vi "CODMn测量数据储存.vi"   [LabVIEW 2016, in "斯坦道CODMn新电路板.lvlib"]
types:
  T1 = enum16{"空闲", "水样测试", "标样核查", "零点核查", "跨度核查", "空白测试", "平行样测试", "加标回收", "空白校准", "标样校准"}
  T2 = enum16{"水样测试", "标样核查", "跨度核查", "零点核查", "空白测试", "平行样测试", "加标回收", "空白校准", "标样校准"}
  T3 = cluster{"时间标识":timestamp, "监测值":sgl, "单位":u16, "数据标识":string, "因子编码":u32, "标样参考值":sgl, "A":sgl, "B":sgl, "K":sgl, "终点滴定数":sgl, "环境温度":sgl, "环境湿度":sgl, "量程":sgl, "加热实时温度":sgl, "X0":sgl, "X^2":sgl, "X":sgl, "B 2":sgl, "跨度值":sgl}
  T4 = enum16{"维护数据", "水样测试", "标样核查", "零点核查", "跨度核查", "空白测试", "平行样测试", "加标回收", "空白校准", "标样校准", "初始化（清洗）"}
  T5 = cluster{"运行模式":enum16{"维护模式", "常规模式", "应急模式", "质控模式"}, "质控频次":enum16{"关闭", "每天", "星期一", "星期二", "星期三", "星期四", "星期五", "星期六", "星期日"}, "空白核查时间":u16, "跨度核查时间":u16, "测量间隔":u16}
  T6 = cluster{"系统时间":timestamp, "工作状态":u16, "测量模式":enum16{"待机", "连续模式", "周期模式", "定点模式", "受控模式", "手动模式"}, "告警代码":u16, "故障代码":u16, "日志代码":u16, "软件版本":u16, "A":sgl, "B":sgl, "K":sgl, "当前滴定数":sgl, "T":sgl, "H":sgl, "id":u16, "flowid":u16, "量程":u16, "加热实时温度":sgl, "当前ORP值":sgl, "运行时间":sgl, "当前步骤剩余时间":sgl, "结束滴定数":sgl, "注射泵保温温度":sgl, "匹配滴定数X0":u16, "X^2":sgl, "X":sgl, "B 2":sgl}
  T7 = cluster{"因子编码":u32, "单位":u16, "标样参考值":sgl, "水样数据时间":timestamp, "水样实测值":sgl, "水样数据标识":string, "标样数据时间":timestamp, "标样实测值":sgl, "标样数据标识":string, "空白数据时间":timestamp, "空白实测值":sgl, "空白数据标识":string, "零点核查数据时间":timestamp, "零点核查实测值":sgl, "零点核查数据标识":string, "跨度核查数据时间":timestamp, "跨度核查实测值":sgl, "跨度核查数据标识":string, "加标回收数据时间":timestamp, "加标回收实测值":sgl, "加标回收数据标识":string, "平行样数据时间":timestamp, "平行样实测值":sgl, "平行样数据标识":string, "F0":sgl, "F1":sgl, "F2":sgl, "F3":sgl, "F4":sgl, "F5":sgl, "F6":sgl, "F7":sgl, "温度":sgl, "湿度":sgl, "X值":sgl, "fidrange":u16}
  T8 = cluster{"跨度值":dbl, "零点标准液浓度":dbl, "跨度标准液浓度":dbl, "标准液标准浓度":dbl}
  T9 = cluster{"公式":cluster{"X^2":dbl, "X":dbl, "B":dbl}, "校准":cluster{"校准？":bool, "校准点1-5":u16, "校准浓度":dbl}}
  T10 = cluster{"测量量程":sgl, "测量检出限":sgl, "测量精度":sgl, "测量间隔":sgl, "消解温度":sgl, "消解时长":sgl, "三项式系数":sgl, "二次多项式系数":sgl, "曲线斜率":sgl, "曲线截距":sgl, "线性相关系数":sgl, "空白校准时间":timestamp, "标样校准时间":timestamp, "测量信号值":sgl, "稀释倍数":sgl, "量程系数":sgl}
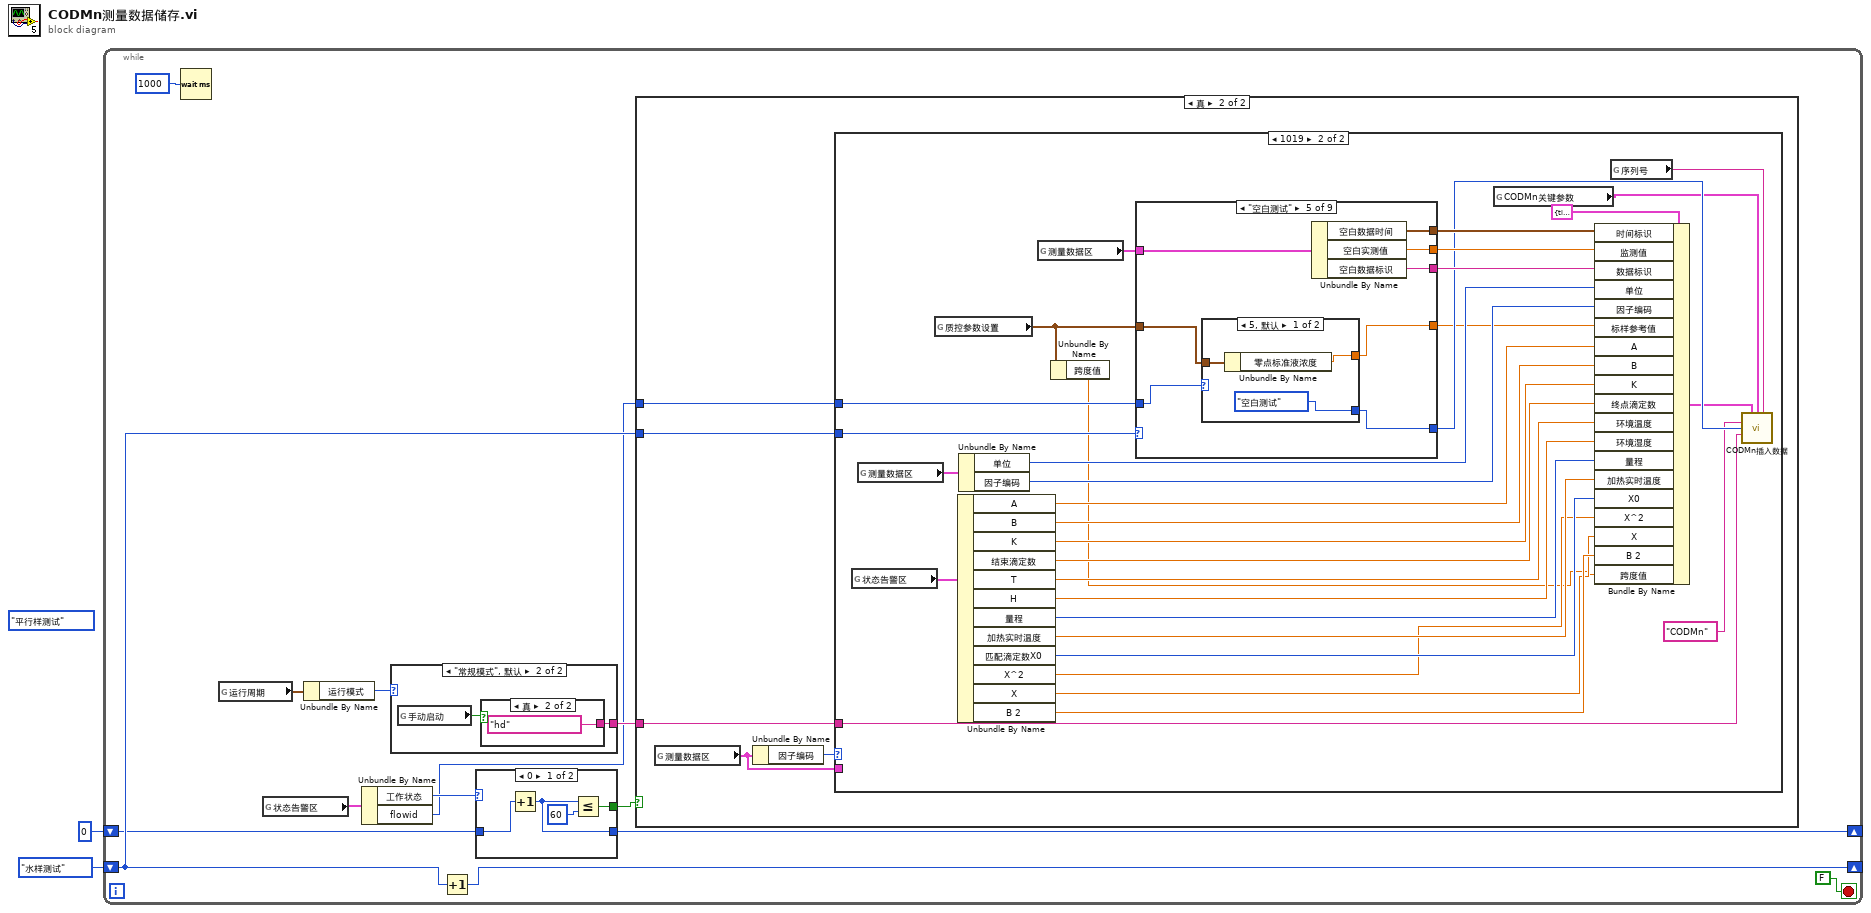
[diagram p0: block diagram]
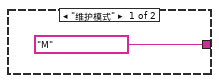
[diagram p2: hidden frame]
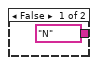
[diagram p3: hidden frame]
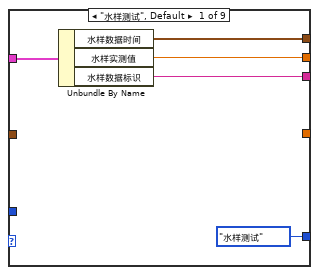
[diagram p7: hidden frame]
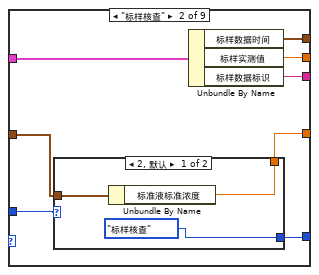
[diagram p8: hidden frame]
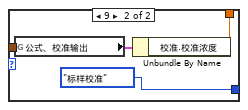
[diagram p9: hidden frame]
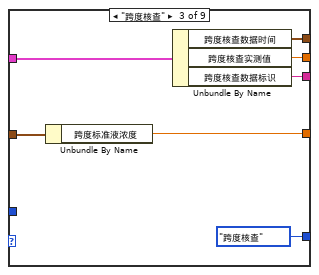
[diagram p10: hidden frame]
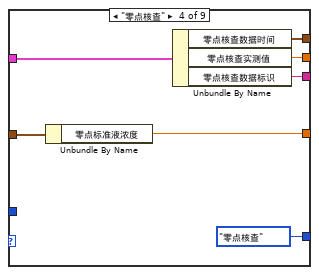
[diagram p11: hidden frame]
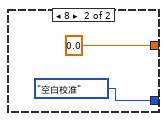
[diagram p12: hidden frame]
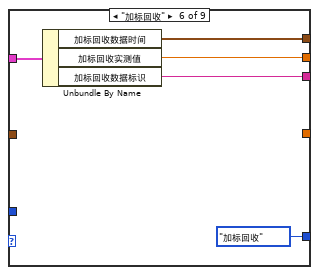
[diagram p13: hidden frame]
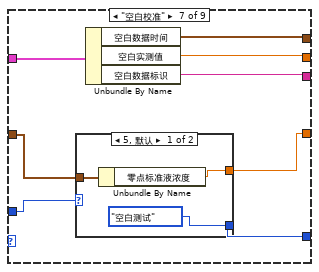
[diagram p14: hidden frame]
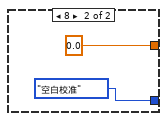
[diagram p15: hidden frame]
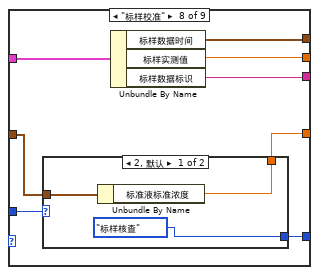
[diagram p16: hidden frame]
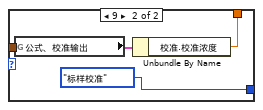
[diagram p17: hidden frame]
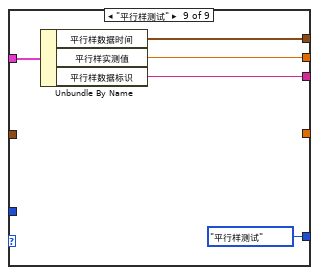
[diagram p18: hidden frame]
diagram:
  (unwired) T1."平行样测试" ("工作状态")
  n1 = while {
    shift-right: [w12] -> _
    shift-left: T2."水样测试" ("测量模式") -> [w11]
    shift-right: [w7] -> _
    shift-left: u32 0 ("等待时间（毫秒）") -> [w8]
    stop <- FALSE stop-if-true
    n2 = Wait (ms)(milliseconds to wait=u32 1000 ("等待时间（毫秒）")) -> ()  [unwired: 1 out]
    n3 = global read "CODMn断电保存全局变量.vi" "运行周期"() -> (w4:T5)
    n4 = global read "VARCODMn全局变量.vi" "状态告警区"() -> (w10:T6)
    n5 = Unbundle By Name(w4) -> ("运行模式"=w3:enum16{"维护模式", "常规模式", "应急模式", "质控模式"})
    n6 = Unbundle By Name(w10) -> ("工作状态"=w9:u16, "flowid"=w5:u16)
    n7 = case shown="\"常规模式\", 默认" w3 {
      tunnel: ["M" ("数据标记表") w18] -> w13
      frame "维护模式" {
      }
      frame "常规模式", Default {
        n8 = global read "VARCODMn全局变量.vi" "手动启动"() -> (w17:bool)
        n9 = case shown="真" w17 {
          tunnel: ["N" ("数据标记表") "hd" ("数据标记表")] -> w18
          frame False {
          }
          frame True {
          }
        }
      }
    }
    n10 = Increment(x=w11) -> (x+1=w12:T2)
    n11 = case shown="0" w9 {
      tunnel: w8 -> [w24 _]
      tunnel: [w23 _] -> w7
      tunnel: [w21 _] -> w6
      frame 0 {
        n12 = Increment(x=w24) -> (x+1=w23:u32)
        n13 = Less Or Equal?(x=w23, y=u32 60) -> (x <= y?=w21:bool)
      }
      frame 1, Default {
      }
    }
    n14 = case shown="真" w6 {
      tunnel: w13 -> [_ w27]
      tunnel: w11 -> [_ w26]
      tunnel: w5 -> [_ w25]
      frame False {
      }
      frame True {
        n15 = global read "VARCODMn全局变量.vi" "测量数据区"() -> (w29:T7)
        n16 = Unbundle By Name(w29) -> ("因子编码"=w28:u32)
        n17 = case shown="1019" w28 {
          tunnel: w29 -> [_ _]
          tunnel: w27 -> [_ w51]
          tunnel: w26 -> [_ w50]
          tunnel: w25 -> [_ w48]
          frame Default {
          }
          frame 1019 {
            n18 = global read "VARCODMn全局变量.vi" "状态告警区"() -> (w47:T6)
            n19 = global read "VARCODMn全局变量.vi" "测量数据区"() -> (w58:T7)
            n20 = global read "CODMn断电保存全局变量.vi" "质控参数设置"() -> (w31:T8)
            n21 = Unbundle By Name(w47) -> ("A"=w40:sgl, "B"=w46:sgl, "K"=w41:sgl, "结束滴定数"=w42:sgl, "T"=w43:sgl, "H"=w39:sgl, "量程"=w44:u16, "加热实时温度"=w45:sgl, "匹配滴定数X0"=w38:u16, "X^2"=w35:sgl, "X"=w36:sgl, "B 2"=w37:sgl)
            n22 = Unbundle By Name(w58) -> ("单位"=w60:u16, "因子编码"=w59:u32)
            n23 = global read "VARCODMn全局变量.vi" "测量数据区"() -> (w61:T7)
            n24 = Unbundle By Name(w31) -> ("跨度值"=w30:dbl)
            n25 = case shown="\"空白测试\"" w50 {
              tunnel: w61 -> [w66 w74 w87 w94 w102 w112 w120 w133 w143]
              tunnel: [w65 w73 w86 w93 w101 w111 w119 w132 w142] -> w54
              tunnel: [w62 w72 w85 w92 w100 w108 w118 w131 w141] -> w55
              tunnel: [w64 w71 w84 w91 w99 w110 w117 w130 w140] -> w56
              tunnel: [T4."水样测试" ("测量模式") w69 T4."跨度核查" ("测量模式") T4."零点核查" ("测量模式") w97 T4."加标回收" ("测量模式") w114 w128 T4."平行样测试" ("测量模式")] -> w53
              tunnel: w31 -> [_ w67 w82 w89 w95 _ w113 w126 _]
              tunnel: [_ w68 w81 w88 w96 _ w116 w127 _] -> w49
              tunnel: w48 -> [_ w70 _ _ w98 _ w115 w129 _]
              frame "水样测试", Default {
                n26 = Unbundle By Name(w66) -> ("水样数据时间"=w65:timestamp, "水样实测值"=w62:sgl, "水样数据标识"=w64:string)
              }
              frame "标样核查" {
                n27 = case shown="2, 默认" w70 {
                  tunnel: [T4."标样核查" ("测量模式") T4."标样校准" ("测量模式")] -> w69
                  tunnel: [w75 w78] -> w68
                  tunnel: w67 -> [w76 _]
                  frame 2, Default {
                    n28 = Unbundle By Name(w76) -> ("标准液标准浓度"=w75:dbl)
                  }
                  frame 9 {
                    n29 = global read "CODMn断电保存全局变量.vi" "公式、校准输出"() -> (w79:T9)
                    n30 = Unbundle By Name(w79) -> ("校准.校准浓度"=w78:dbl)
                  }
                }
                n31 = Unbundle By Name(w74) -> ("标样数据时间"=w73:timestamp, "标样实测值"=w72:sgl, "标样数据标识"=w71:string)
              }
              frame "跨度核查" {
                n32 = Unbundle By Name(w82) -> ("跨度标准液浓度"=w81:dbl)
                n33 = Unbundle By Name(w87) -> ("跨度核查数据时间"=w86:timestamp, "跨度核查实测值"=w85:sgl, "跨度核查数据标识"=w84:string)
              }
              frame "零点核查" {
                n34 = Unbundle By Name(w89) -> ("零点标准液浓度"=w88:dbl)
                n35 = Unbundle By Name(w94) -> ("零点核查数据时间"=w93:timestamp, "零点核查实测值"=w92:sgl, "零点核查数据标识"=w91:string)
              }
              frame "空白测试" {
                n36 = case shown="5, 默认" w98 {
                  tunnel: [T4."空白测试" ("测量模式") T4."空白校准" ("测量模式")] -> w97
                  tunnel: [w103 0.0 ("零点标准液浓度")] -> w96
                  tunnel: w95 -> [w104 _]
                  frame 5, Default {
                    n37 = Unbundle By Name(w104) -> ("零点标准液浓度"=w103:dbl)
                  }
                  frame 8 {
                  }
                }
                n38 = Unbundle By Name(w102) -> ("空白数据时间"=w101:timestamp, "空白实测值"=w100:sgl, "空白数据标识"=w99:string)
              }
              frame "加标回收" {
                n39 = Unbundle By Name(w112) -> ("加标回收数据时间"=w111:timestamp, "加标回收实测值"=w108:sgl, "加标回收数据标识"=w110:string)
              }
              frame "空白校准" {
                n40 = case shown="5, 默认" w115 {
                  tunnel: [T4."空白测试" ("测量模式") T4."空白校准" ("测量模式")] -> w114
                  tunnel: [w121 0.0 ("零点标准液浓度")] -> w116
                  tunnel: w113 -> [w122 _]
                  frame 5, Default {
                    n41 = Unbundle By Name(w122) -> ("零点标准液浓度"=w121:dbl)
                  }
                  frame 8 {
                  }
                }
                n42 = Unbundle By Name(w120) -> ("空白数据时间"=w119:timestamp, "空白实测值"=w118:sgl, "空白数据标识"=w117:string)
              }
              frame "标样校准" {
                n43 = case shown="2, 默认" w129 {
                  tunnel: [T4."标样核查" ("测量模式") T4."标样校准" ("测量模式")] -> w128
                  tunnel: [w134 w137] -> w127
                  tunnel: w126 -> [w135 _]
                  frame 2, Default {
                    n44 = Unbundle By Name(w135) -> ("标准液标准浓度"=w134:dbl)
                  }
                  frame 9 {
                    n45 = global read "CODMn断电保存全局变量.vi" "公式、校准输出"() -> (w138:T9)
                    n46 = Unbundle By Name(w138) -> ("校准.校准浓度"=w137:dbl)
                  }
                }
                n47 = Unbundle By Name(w133) -> ("标样数据时间"=w132:timestamp, "标样实测值"=w131:sgl, "标样数据标识"=w130:string)
              }
              frame "平行样测试" {
                n48 = Unbundle By Name(w143) -> ("平行样数据时间"=w142:timestamp, "平行样实测值"=w141:sgl, "平行样数据标识"=w140:string)
              }
            }
            n49 = global read "CODMn断电保存全局变量.vi" "CODMn关键参数"() -> (w34:T10)
            n50 = Bundle By Name(cluster=T3 {"时间标识"=timestamp(0 s since 1904-01-01), "监测值"=0.0, "单位"=0, "数据标识"="", "因子编码"=0, "标样参考值"=0.0, "A"=0.0, "B"=0.0, "K"=0.0, "终点滴定数"=0.0, "环境温度"=0.0, "环境湿度"=0.0, "量程"=0.0, "加热实时温度"=0.0, "X0"=0.0, "X^2"=0.0, "X"=0.0, "B 2"=0.0, "跨度值"=0.0} ("data"), "时间标识"=w54, "监测值"=w55, "数据标识"=w56, "单位"=w60, "因子编码"=w59, "标样参考值"=w49, "A"=w40, "B"=w46, "K"=w41, "终点滴定数"=w42, "环境温度"=w43, "环境湿度"=w39, "量程"=w44, "加热实时温度"=w45, "X0"=w38, "X^2"=w35, "X"=w36, "B 2"=w37, "跨度值"=w30) -> (w32:T3)
            n51 = global read "VARCODMn全局变量.vi" "序列号"() -> (w57:string)
            n52 = call "CODMn插入数据.vi"("data"=w32, "CODMn关键参数"=w34, "SN"=w57, "table"="CODMn", "测量模式"=w53, "数据类型"=w51) -> ()  [unwired: 9 in, 1 out]
          }
        }
      }
    }
  }
